vi "ConfigureChannelProperties.vi"(8 "error in (no error)":errorcluster, 9 "Sampling Rate":dbl format="%#_13g", 10 "Filtered Channels (in acquisition order)":T4[](array[typedef])) -> (0 "error out":errorcluster, 2 "Channel Config X31":T2 {"InputConfig" items=["AC Coupled", "DC Coupled", "IEPE AC Coupled"]}, 3 "Sampling Info":T1={"Number of Channels"=4, "Sampling Rate"=4.0, "Channels"=[], "Units"=[], "Offsets"=[]})   [LabVIEW 2017, in "McsaFpgaAcquisition.lvlib"]
uses:
  <vilib>/addons/InsightCM/Devices/Shared/Mcsa/McsaFpgaAcquisition/McsaFpgaAcquisition.lvlib
  <vilib>/addons/InsightCM/MessageBus/Base/controls/R2_Channel.ctl
  <vilib>/addons/InsightCM/MessageBus/Base/controls/KeyValuePair.ctl
  <vilib>/addons/InsightCM/MessageBus/Base/controls/Metric.ctl
  <vilib>/addons/InsightCM/Devices/Shared/Cms/CmsAcquisition/controls/FixedSizeArrays.ctl
  <vilib>/LabVIEW Targets/FPGA/cRIO/shared/nicrio_ModuleControls/nicrio_cRIO-9232_ConfigModeRing.ctl
  <vilib>/addons/InsightCM/Devices/Shared/Cms/cRIOWfmAcq/subVIs/RIO Wfm Cust Ctrls/rwfm_SamplingInfo.ctl
  <vilib>/addons/InsightCM/Devices/Shared/Cms/cRIOWfmAcq/cRIOWfmLib.lvlib
  <vilib>/addons/InsightCM/Utilities/PropertyHelpers/PropertyHelpers.lvlib
  <vilib>/addons/InsightCM/Devices/Shared/Cms/CmsAcquisition/CmsAcquisition.lvlib
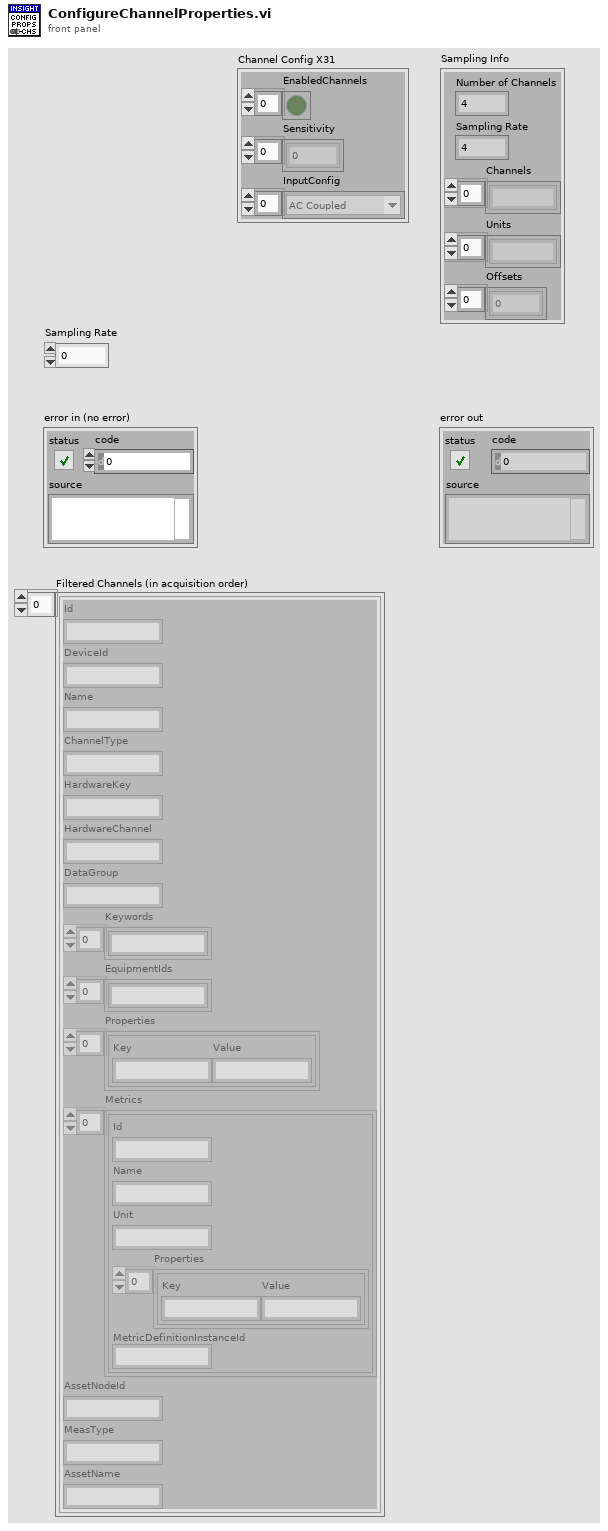
[diagram p1: front panel]
types:
  T1 = typedef "cRIOWfmLib.lvlib/rwfm_SamplingInfo.ctl" = cluster{"Number of Channels":i32, "Sampling Rate":dbl, "Channels":string[], "Units":string[], "Offsets":sgl[]}
  T2 = typedef "CmsAcquisition.lvlib/FixedSizeArrays.ctl" = cluster{"EnabledChannels":bool[], "Sensitivity":dbl[], "InputConfig":T3[]}
  T3 = typedef "nicrio_cRIO-9232_ConfigModeRing.ctl" = u8
  T4 = typedef "R2_Channel.ctl" = cluster{"Id":string, "DeviceId":string, "Name":string, "ChannelType":string, "HardwareKey":string, "HardwareChannel":string, "DataGroup":string, "Keywords":string[], "EquipmentIds":string[], "Properties":T5[], "Metrics":T6[], "AssetNodeId":string, "MeasType":string, "AssetName":string}
  T5 = typedef "KeyValuePair.ctl" = cluster{"Key":string, "Value":string}
  T6 = typedef "Metric.ctl" = cluster{"Id":string, "Name":string, "Unit":string, "Properties":T5[], "MetricDefinitionInstanceId":string}
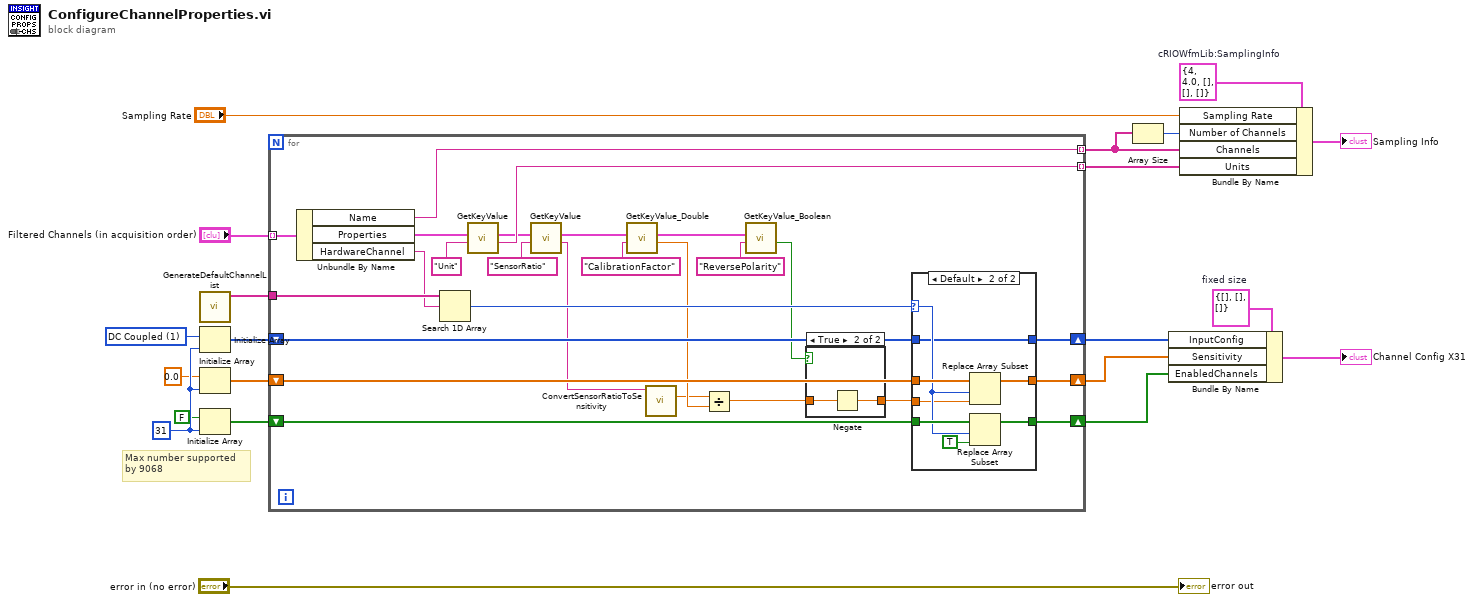
[diagram p0: block diagram]
diagram:
  w8 = T1 {"Number of Channels"=4, "Sampling Rate"=4.0, "Channels"=[], "Units"=[], "Offsets"=[]}  # cRIOWfmLib:SamplingInfo
  w16 = T2 {"EnabledChannels"=[], "Sensitivity"=[], "InputConfig"=[]}  # fixed size
  w12 = T3 1 items=["AC Coupled", "DC Coupled", "IEPE AC Coupled"] ("Input_Configuration")
  w13 = 31 ("dimension size")
  # "Max number supported\nby 9068"
  n1 = call <vilib>:"GenerateDefaultChannelList.vi"() -> ("default channel list"=w1:string[])  [unwired: 11 in]
  n2 = Initialize Array(w12, w13) -> (w15:T3[])
  n3 = Initialize Array(0.0 ("value"), w13) -> (w14:dbl[])
  n4 = Initialize Array(FALSE, w13) -> (w10:bool[])
  n5 = for {
    tunnel: "Filtered Channels (in acquisition order)" -> [w41] mode=indexing
    shift-right: [w46] -> w19
    shift-left: w10 -> [w47]
    shift-right: [w44] -> w18
    shift-left: w14 -> [w45]
    shift-right: [w42] -> w17
    shift-left: w15 -> [w43]
    tunnel: w1 -> [w40]
    tunnel: [w38] -> w5 mode=indexing
    tunnel: [w34] -> w7 mode=indexing
    n6 = Unbundle By Name(w41) -> ("Name"=w38:string, "Properties"=w36:T5[], "HardwareChannel"=w39:string)
    n7 = Search 1D Array(1D array=w40, element=w39) -> (index of element=w37:i32)  [unwired: 1 in]
    n8 = call <vilib>:"GetKeyValue.vi"("key"="Unit" ("name"), "key value pairs"=w36) -> ("value"=w34:string, "key value pairs out"=w33:T5[])  [unwired: 7 in, 1 out]
    n9 = call <vilib>:"GetKeyValue.vi"("key"="SensorRatio" ("name"), "key value pairs"=w33) -> ("value"=w23:string, "key value pairs out"=w30:T5[])  [unwired: 7 in, 1 out]
    n10 = call <vilib>:"GetKeyValue_Double.vi"("key"="CalibrationFactor" ("name"), "key value pairs"=w30) -> ("value"=w24:dbl, "key value pairs out"=w28:T5[])  [unwired: 7 in, 1 out]
    n11 = call <vilib>:"ConvertSensorRatioToSensitivity.vi"("sensor ratio"=w23) -> ("sensitivity"=w22:dbl)  [unwired: 10 in]
    n12 = Divide(x=w22, y=w24) -> (x/y=w25:dbl)
    n13 = call <vilib>:"GetKeyValue_Boolean.vi"("key"="ReversePolarity" ("name"), "key value pairs"=w28) -> ("value"=w27:bool)  [unwired: 7 in, 2 out]
    n14 = case shown="True" w27 {
      tunnel: [w48 w50] -> w26
      tunnel: w25 -> [w48 w49]
      frame False {
      }
      frame True {
        n15 = Negate(x=w49) -> (-x=w50:dbl)
      }
    }
    n16 = case shown="Default" w37 {
      selector: w37 -> [_ w57]
      tunnel: w47 -> [w53 w61]
      tunnel: [w53 w59] -> w46
      tunnel: w45 -> [w51 w58]
      tunnel: [w51 w56] -> w44
      tunnel: w43 -> [w52 w54]
      tunnel: [w52 w54] -> w42
      tunnel: w26 -> [_ w55]
      frame -1 {
      }
      frame Default {
        n17 = Replace Array Subset(array=w58, new element=w55, index=w57) -> (w56:dbl[])
        n18 = Replace Array Subset(array=w61, new element=TRUE, index=w57) -> (w59:bool[])
      }
    }
  }
  n19 = Array Size(array=w5) -> (size(s)=w4:i32)
  n20 = Bundle By Name(cluster=w16, "InputConfig"=w17, "Sensitivity"=w18, "EnabledChannels"=w19) -> (→"Channel Config X31":T2)
  n21 = Bundle By Name(cluster=w8, "Sampling Rate"="Sampling Rate", "Number of Channels"=w4, "Channels"=w5, "Units"=w7) -> (→"Sampling Info":T1)
  "error out" <- "error in (no error)"
